vi "XVA-DSE6_defaut.vi"(8 "err in":errorcluster, 10 "tmax":dbl, 11 "paramètres":T17) -> (0 "err out":errorcluster, 2 "Graphe LN f et F":cluster{dbl[], dbl[]}[](graph) caption="Densité de Probabilité f et Fonction de Répartition F", 3 "X-VA (s)":T1)   [LabVIEW 2010, in "lv_04.lvlib"]
uses:
  lv_02/p_5E6_Lexp.ctl
  commandes/cX.ctl
  commandes/cSTA_varid.ctl
  commandes/c_TDMS_ch_variable.ctl
  commandes/c_TDMS_ch_donnees.ctl
  commandes/c0-var-n.ctl
  commandes/cSTA_num_do_cr.ctl
  commandes/c02-do-num.ctl
  commandes/c04-stat-num.ctl
  commandes/cSTA_txt_do_cr.ctl
  commandes/c02-do-txt.ctl
  commandes/c04-stat-txt.ctl
  commandes/cSTA_dist.ctl
  commandes/c03-dist-S.ctl
  commandes/c0-dist-xy.ctl
  commandes/c03-dist-T.ctl
  commandes/c03-dist-SPC.ctl
  XVA-DSE6-dist.vi
  lv_04.lvlib
  lv_02/lv_02.lvlib
panel:
  # "Loi Exponentielle"
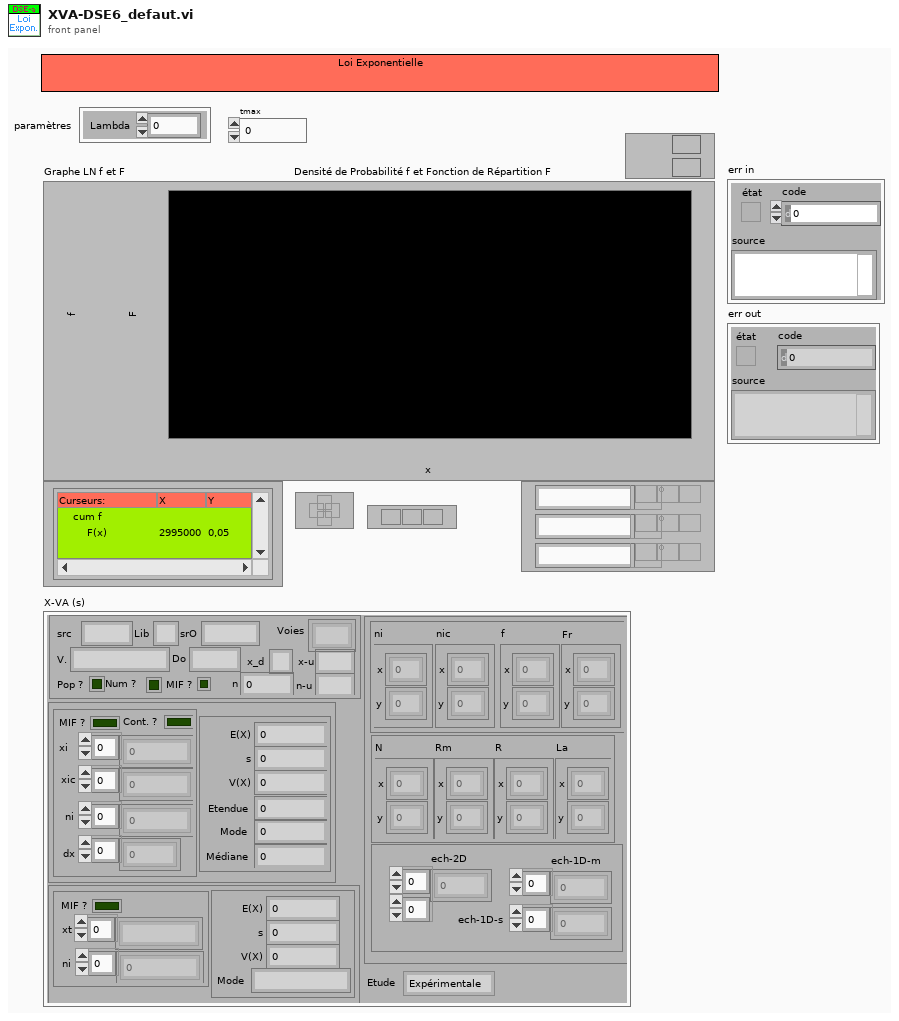
[diagram p1: front panel]
types:
  T1 = typedef "lv_04.lvlib/cX.ctl" = cluster{"src":T2, "num":T6, "txt":T9, "dist":T12, "Etude":enum16{"Expérimentale", "Modèle"}}
  T2 = typedef "lv_04.lvlib/cSTA_varid.ctl" = cluster{"src":string, "Lib":string, "srO":string, "V.":T3, "Voies":string[], "Do":T4, "n":T5, "Num ?":bool, "Pop ?":bool, "x_d":string, "x-u":string, "n-u":string, "MIF ?":bool}
  T3 = typedef "lv_04.lvlib/c_TDMS_ch_variable.ctl" = string
  T4 = typedef "lv_04.lvlib/c_TDMS_ch_donnees.ctl" = string
  T5 = typedef "lv_04.lvlib/c0-var-n.ctl" = i32
  T6 = typedef "lv_04.lvlib/cSTA_num_do_cr.ctl" = cluster{"do":T7, "sta":T8}
  T7 = typedef "lv_04.lvlib/c02-do-num.ctl" = cluster{"MIF ?":bool, "Cont. ?":bool, "xi":dbl[], "xic":dbl[], "ni":u32[], "dx":dbl[]}
  T8 = typedef "lv_04.lvlib/c04-stat-num.ctl" = cluster{"E(X)":dbl, "s":dbl, "V(X) ":dbl, "Etendue":dbl, "Mode":dbl, "Médiane":dbl}
  T9 = typedef "lv_04.lvlib/cSTA_txt_do_cr.ctl" = cluster{"do":T10, "sta":T11}
  T10 = typedef "lv_04.lvlib/c02-do-txt.ctl" = cluster{"xt":string[], "ni":dbl[], "MIF ?":bool}
  T11 = typedef "lv_04.lvlib/c04-stat-txt.ctl" = cluster{"E(X)":dbl, "s":dbl, "V(X) ":dbl, "Mode":string}
  T12 = typedef "lv_04.lvlib/cSTA_dist.ctl" = cluster{"S":T13, "T":T15, "spc":T16}
  T13 = typedef "lv_04.lvlib/c03-dist-S.ctl" = cluster{"nic":T14, "f":T14, "Fr":T14, "ni":T14}
  T14 = typedef "lv_04.lvlib/c0-dist-xy.ctl" = cluster{"x":dbl[], "y":dbl[]}
  T15 = typedef "lv_04.lvlib/c03-dist-T.ctl" = cluster{"N":T14, "Rm":T14, "R":T14, "La":T14}
  T16 = typedef "lv_04.lvlib/c03-dist-SPC.ctl" = cluster{"ech-2D":dbl[][], "ech-1D-m":dbl[], "ech-1D-s":dbl[]}
  T17 = typedef "lv_02.lvlib/p_5E6_Lexp.ctl" = cluster{"Lambda":dbl}
  T18 = typedef "lv_01.lvlib/do_serie-c.ctl" = cluster{"X":dbl[], "par":cluster{"x_deb":dbl, "Pas":dbl, "Nb":dbl}}
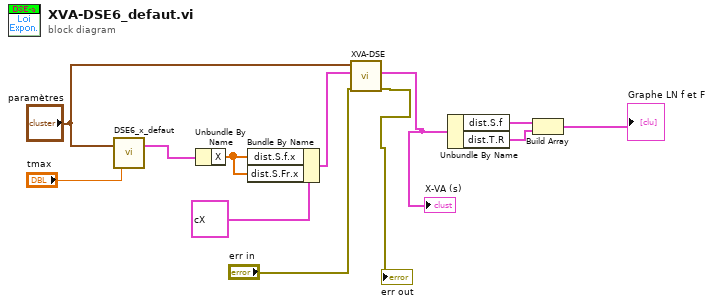
[diagram p0: block diagram]
diagram:
  n1 = call "DSE6_x_defaut.vi"("tmax"="tmax", "Loi Expo."="paramètres") -> ("X (Défaut)"=w3:T18)  [unwired: 1 in]
  n2 = Unbundle By Name(w3) -> ("X"=w11:dbl[])
  n3 = Bundle By Name(cluster=T1 {"src"={"src"="", "Lib"="", "srO"="", "V."="", "Voies"=[], "Do"="", "n"=0, "Num ?"=FALSE, "Pop ?"=FALSE, "x_d"="", "x-u"="", "n-u"="", "MIF ?"=FALSE}, "num"={"do"={"MIF ?"=FALSE, "Cont. ?"=FALSE, "xi"=[], "xic"=[], "ni"=[], "dx"=[]}, "sta"={"E(X)"=0.0, "s"=0.0, "V(X) "=0.0, "Etendue"=0.0, "Mode"=0.0, "Médiane"=0.0}}, "txt"={"do"={"xt"=[], "ni"=[], "MIF ?"=FALSE}, "sta"={"E(X)"=0.0, "s"=0.0, "V(X) "=0.0, "Mode"=""}}, "dist"={"S"={"nic"={"x"=[], "y"=[]}, "f"={"x"=[], "y"=[]}, "Fr"={"x"=[], "y"=[]}, "ni"={"x"=[], "y"=[]}}, "T"={"N"={"x"=[], "y"=[]}, "Rm"={"x"=[], "y"=[]}, "R"={"x"=[], "y"=[]}, "La"={"x"=[], "y"=[]}}, "spc"={"ech-2D"=[], "ech-1D-m"=[], "ech-1D-s"=[]}}, "Etude"=enum."Expérimentale"} ("cXB (s)"), "dist.S.f.x"=w11, "dist.S.Fr.x"=w11) -> (w7:T1)
  n4 = call-poly "XVA-DSE.vi"("err in"="err in", "X-VA (e)"=w7, "p_LExp"="paramètres") -> ("err out"=→"err out":errorcluster, "VA (s)"=w4:T1)  [unwired: 6 in, 1 out]
  "X-VA (s)" <- w4
  n5 = Unbundle By Name(w4) -> ("dist.S.f"=w10:T14, "dist.T.R"=w9:T14)
  n6 = Build Array(w10, w9) -> (→"Graphe LN f et F":T14[])
